vi "Fahrenheit to Celsius.vi"() -> ()   [LabVIEW 2023]
panel:
  out "Celsius":dbl(slide) scale=0.0..1000.0
  in  "Fahrenheit":dbl(slide) scale=0.0..2000.0
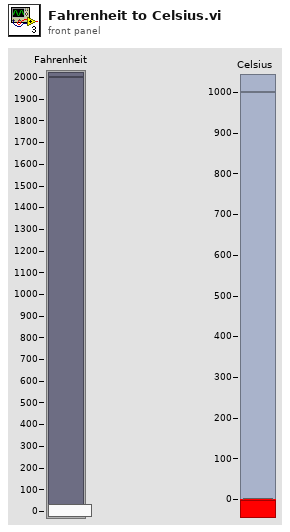
[diagram p1: front panel]
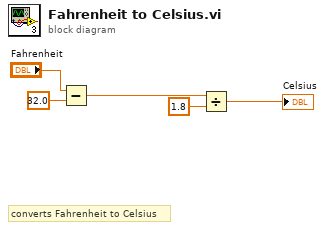
[diagram p0: block diagram]
diagram:
  # "converts Fahrenheit to Celsius"
  n1 = Subtract(x="Fahrenheit", y=32.0) -> (x-y=w5:dbl)
  n2 = Divide(x=w5, y=1.8) -> (x/y=→"Celsius":dbl)
